vi "Write String.vi"(7 "Channel Name":string, 8 "error in (no error)":errorcluster, 9 "Data Value":dbl, 10 "Bus In":refnum<class "Bus.lvclass">, 11 "Output in":refnum<class "Output.lvclass">) -> (0 "error out":errorcluster, 2 "Bus Out":refnum<class "Bus.lvclass">, 3 "Output out":refnum<class "Output.lvclass">)   [LabVIEW 2018, in "Output.lvclass"]
doc: "Otput.lvclass:Write String.vi\n\nThis is the template for the Write String VI for the Output class.\n\nInstrument Communication Module Version 1.0\nOctober, 2020 Original Code Consulting Davita Bird\n www.originalcode.com"
uses:
  Output.lvclass
  Bus/Bus.lvclass
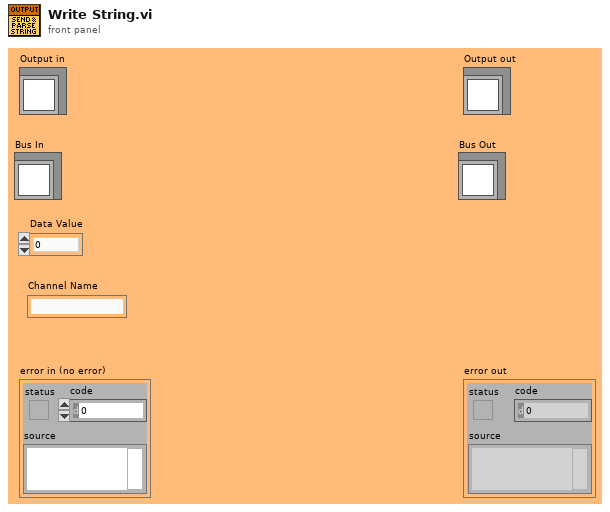
[diagram p1: front panel]
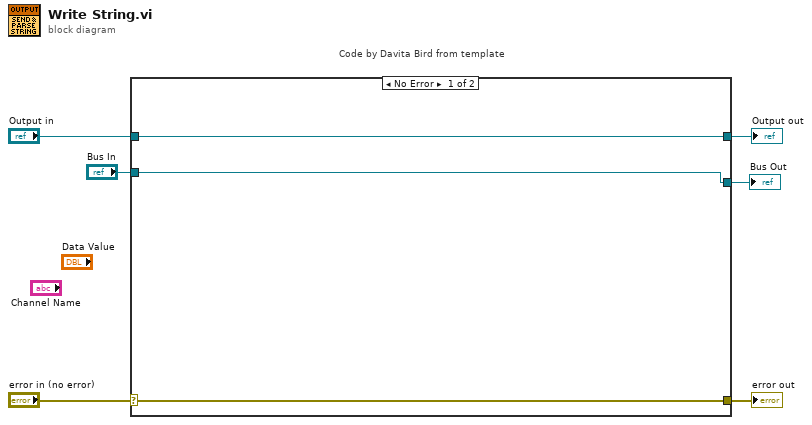
[diagram p0: block diagram]
diagram:
  n1 = case "Code by Davita Bird from template" shown="No Error" "error in (no error)" {
    selector: "error in (no error)" -> [w8 w12]
    tunnel: [w8 w12] -> w5
    tunnel: [w9 w11] -> w3
    tunnel: "Output in" -> [w9 w11]
    tunnel: "Bus In" -> [w7 w10]
    tunnel: [w7 w10] -> w1
    frame No Error {
    }
    frame Error {
    }
  }
  "error out" <- w5
  "Output out" <- w3
  "Bus Out" <- w1
